vi "kinectRead [BodyFrame].vi"(6 "Coordinate Space":enum16{"Color Space", "Depth Space"}(ring), 8 "error in (no error)":errorcluster, 9 "Timeout (ms)":i32=5000, 11 "KinectSensor References in":T2) -> (0 "error out":errorcluster, 2 "Body Data":T1[](array[typedef]) {"LeanTrackingState" items=["NotTracked", "Inferred", "Tracked"]; "HandRightState" items=["Unknown", "NotTracked", "Open", "Closed", "Lasso"]; "HandRightConfidence" items=["Low", "High"]; "HandLeftState" items=["Unknown", "NotTracked", "Open", "Closed", "Lasso"]; "HandLeftConfidence" items=["Low", "High"]; "ClippedEdges" items=["None"=0, "Right"=1, "Left"=2, "Top"=4, "Bottom"=8]}, 3 "KinectSensor References out":T2)   [LabVIEW 2014]
uses:
  controls/KinectSensor References.ctl
  Microsoft.Kinect
  C:/github/labviewhacker/LVH-KinectOne/LabVIEW/vi.lib/LabVIEW Hacker/KinectOne/support/BodyFrameDataInterface.dll
  BodyFrameDataInterface.dll
  controls/BodyData.ctl
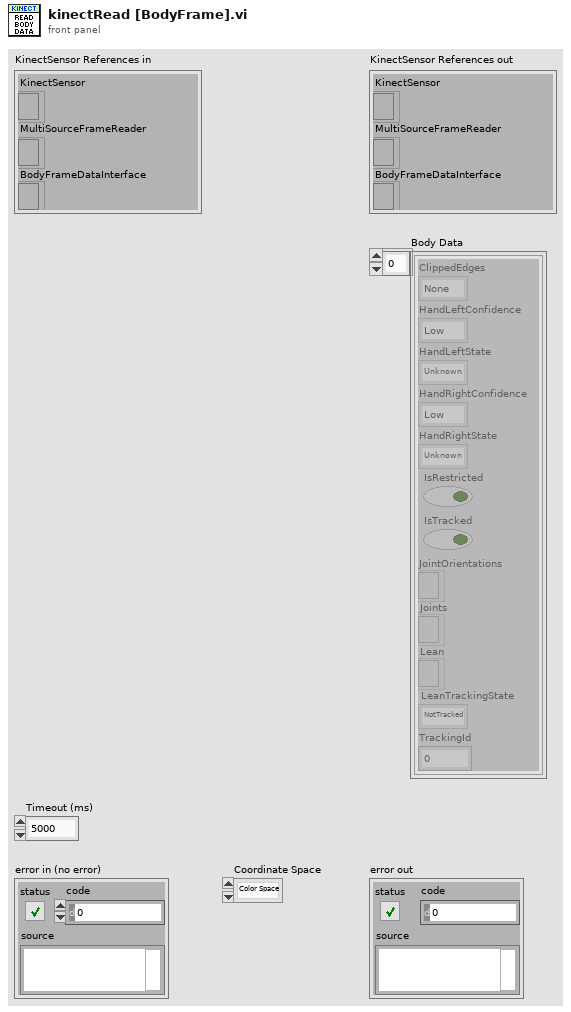
[diagram p1: front panel]
types:
  T1 = typedef "BodyData.ctl" = cluster{"ClippedEdges":i32, "HandLeftConfidence":i32, "HandLeftState":i32, "HandRightConfidence":i32, "HandRightState":i32, "IsRestricted":bool, "IsTracked":bool, "JointOrientations":refnum<k24>, "Joints":refnum<k24>, "Lean":refnum<k24>, "LeanTrackingState":i32, "TrackingId":u64}
  T2 = typedef "KinectSensor References.ctl" = cluster{"KinectSensor":refnum<k24>, "MultiSourceFrameReader":refnum<k24>, "BodyFrameDataInterface":refnum<k24>}
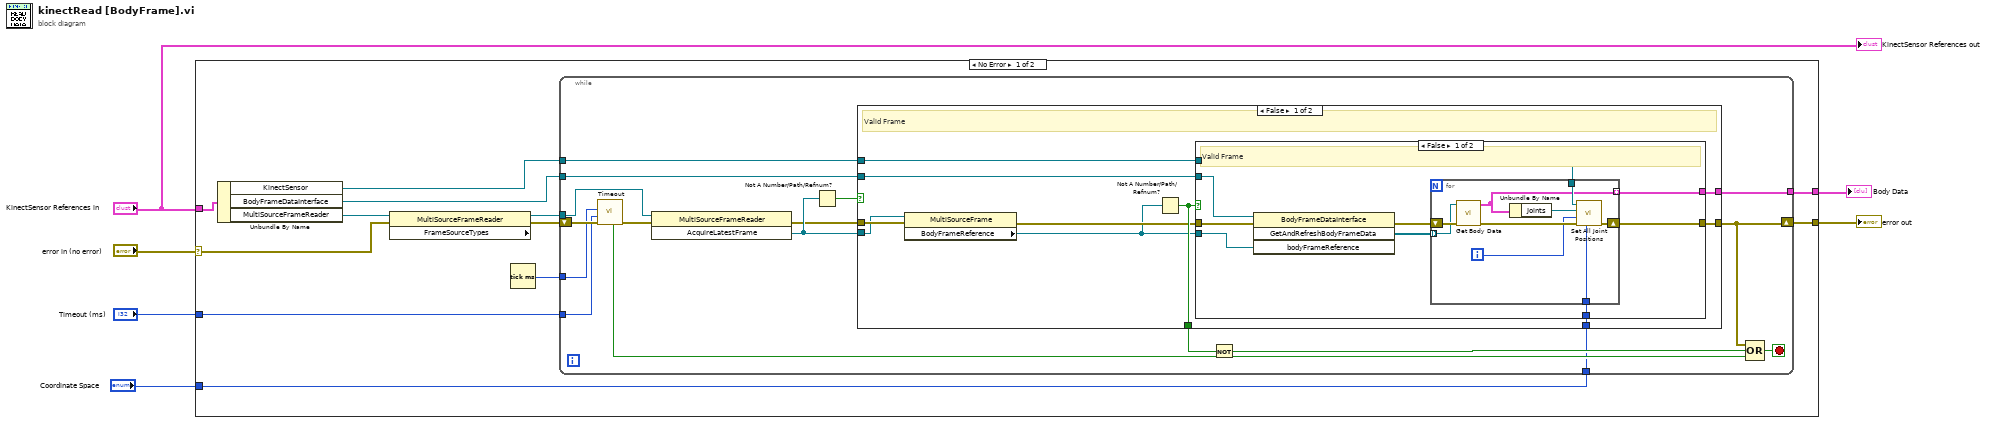
[diagram p0: block diagram]
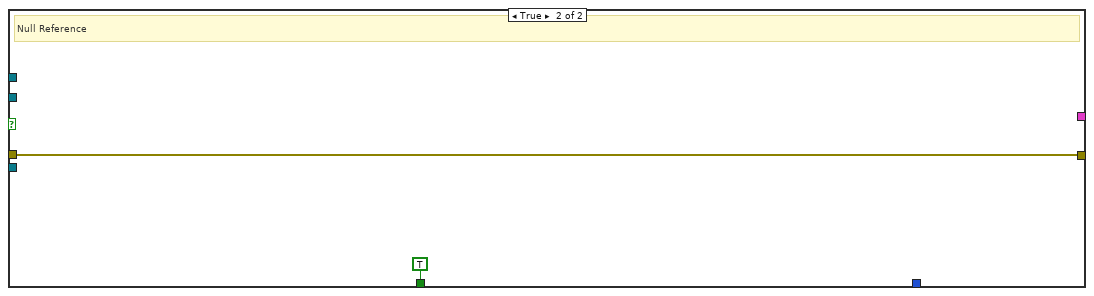
[diagram p3: hidden frame]
diagram:
  n1 = case shown="No Error" "error in (no error)" {
    selector: "error in (no error)" -> [w9 w67]
    tunnel: "KinectSensor References in" -> [w15 _]
    tunnel: [w14 w67] -> w5
    tunnel: [w13 _] -> w4
    tunnel: "Timeout (ms)" -> [w10 _]
    tunnel: "Coordinate Space" -> [w7 _]
    frame No Error {
      n2 = Unbundle By Name(w15) -> ("KinectSensor"=w8:refnum<k24>, "BodyFrameDataInterface"=w12:refnum<k24>, "MultiSourceFrameReader"=w16:refnum<k24>)
      n3 = property class="MultiSourceFrameReader" props=["FrameSourceTypes"](reference=w16, error in=w9) -> (reference out=w18:refnum<k24>, error out=w17:errorcluster)  [unwired: 1 out]
      n4 = Tick Count (ms)() -> (millisecond timer value=w11:u32)
      n5 = while {
        tunnel: w18 -> [w30]
        shift-right: [w25] -> w14
        shift-left: w17 -> [w29]
        tunnel: [w32] -> w13
        tunnel: w12 -> [w31]
        tunnel: w11 -> [w27]
        tunnel: w10 -> [w26]
        tunnel: w8 -> [w20]
        tunnel: w7 -> [w19]
        stop <- w24 stop-if-true
        n6 = call "Timeout.vi"("error in (no error)"=w29, "Timeout (ms)"=w26, "Start Time"=w27) -> ("error out"=w28:errorcluster, "Timeout?"=w21:bool)  [unwired: 7 in]
        n7 = invoke class="MultiSourceFrameReader" method="AcquireLatestFrame"(reference=w30, error in=w28) -> (error out=w34:errorcluster, "AcquireLatestFrame"=w35:refnum<k24>)  [unwired: 1 in, 1 out]
        n8 = Not A Number/Path/Refnum?(number/path/refnum=w35) -> (NaN/Path/Refnum?=w33:bool)
        n9 = case shown="False" w33 {
          tunnel: w34 -> [w45 w65]
          tunnel: w35 -> [w42 _]
          tunnel: [w44 w65] -> w25
          tunnel: [w43 TRUE] -> w23
          tunnel: w31 -> [w41 _]
          tunnel: [w40 _] -> w32
          tunnel: w20 -> [w37 _]
          tunnel: w19 -> [w36 _]
          frame False {
            # "Valid Frame"
            n10 = property class="MultiSourceFrame"(reference=w42, error in=w45) -> (error out=w39:errorcluster, "BodyFrameReference"=w38:refnum<k24>)  [unwired: 1 out]
            n11 = Not A Number/Path/Refnum?(number/path/refnum=w38) -> (NaN/Path/Refnum?=w43:bool)
            n12 = case shown="False" w43 {
              tunnel: [w48 w64] -> w44
              tunnel: w41 -> [w52 _]
              tunnel: [w51 _] -> w40
              tunnel: w39 -> [w49 w64]
              tunnel: w38 -> [w50 _]
              tunnel: w37 -> [w47 _]
              tunnel: w36 -> [w46 _]
              frame False {
                # "Valid Frame"
                n13 = invoke class="BodyFrameDataInterface" method="GetAndRefreshBodyFrameData"(reference=w52, error in=w49, "bodyFrameReference"=w50) -> (error out=w53:errorcluster, "GetAndRefreshBodyFrameData"=w54:refnum<k24>[])  [unwired: 1 in, 2 out]
                n14 = for {
                  tunnel: w54 -> [w62] mode=indexing
                  shift-right: [w61] -> w48
                  shift-left: w53 -> [w63]
                  tunnel: [w56] -> w51 mode=indexing
                  tunnel: w47 -> [w57]
                  tunnel: w46 -> [w55]
                  i -> [w59]
                  n15 = call "Get Body Data.vi"("error in (no error)"=w63, "Body Reference"=w62) -> ("error out"=w60:errorcluster, "BodyData"=w56:T1)  [unwired: 8 in]
                  n16 = Unbundle By Name(w56) -> ("Joints"=w58:refnum<k24>)
                  n17 = call "Set All Joint Positions.vi"("Coordinate Space"=w55, "error in (no error)"=w60, "Body Index"=w59, "Joints"=w58, "KinectSensor Reference"=w57) -> ("error out"=w61:errorcluster)  [unwired: 6 in]
                }
              }
              frame True {
                # "Null Reference"
              }
            }
          }
          frame True {
            # "Null Reference"
          }
        }
        n18 = Not(x=w23) -> (.not. x?=w22:bool)
        n19 = Compound Arithmetic op=OR(w25, w22, w21) -> (w24:bool)
      }
    }
    frame Error {
    }
  }
  "error out" <- w5
  "Body Data" <- w4
  "KinectSensor References out" <- "KinectSensor References in"
